vi "Segway - Segue linha suave.vi"() -> ()   [LabVIEW 2016]
uses:
  <vilib>/NXT/Block Support/NXT_InputPort.ctl
  <vilib>/NXT/Subs/MotorOutput.ctl
  <vilib>/NXT/Block Support/NXT_TimerIndex.ctl
  <vilib>/NXT/Block Support/NXT_OutputPort.ctl
  <vilib>/NXT/Dual Mode Library/Waits/Wait_Num.vi
  <vilib>/NXT/Dual Mode Library/Sensors/EV3_Gyro_Reset.vi
  <vilib>/NXT/Dual Mode Library/Motors/ResetMotor.vi
  <vilib>/NXT/Dual Mode Library/Display/drawNumber.vi
  <vilib>/NXT/Dual Mode Library/Sensors/EV3_Color_Reflect.vi
  <vilib>/NXT/Dual Mode Library/Sensors/EV3_Gyro_Rate.vi
  <vilib>/NXT/Dual Mode Library/Motors/Rotation.vi
  <vilib>/NXT/NXTIO Xnodes/NXTIONodeSubVIs/NXTMoveMotors.vi
  <vilib>/NXT/NXTIO Xnodes/AddressXNode/NXTIOAddress.xnode
  <vilib>/NXT/NXTIO Xnodes/NXTIOXNode/NXTIO.xnode
  <vilib>/NXT/Subs/LVHSConnector.ctl
  <vilib>/NXT/LegoClasses/BrickReference/BrickReference.lvclass
panel:
  out "Seguidor E":dbl
  out "Seguidor D":dbl
  in  "stop":bool
  out "e":dbl
  out "Waveform Chart 2":dbl(graph)
  out "b":dbl
  out "a":dbl
  in  "dt_program_flow":dbl
  out "dt":dbl
  out "timer_time":dbl
  out "EncSum":dbl
  out "VelAngRoda2":dbl(graph)
  out "PosAngRoda2":dbl(graph)
  out "PosAngCorpo2":dbl(graph)
  out "VelAngCorpo2":dbl(graph)
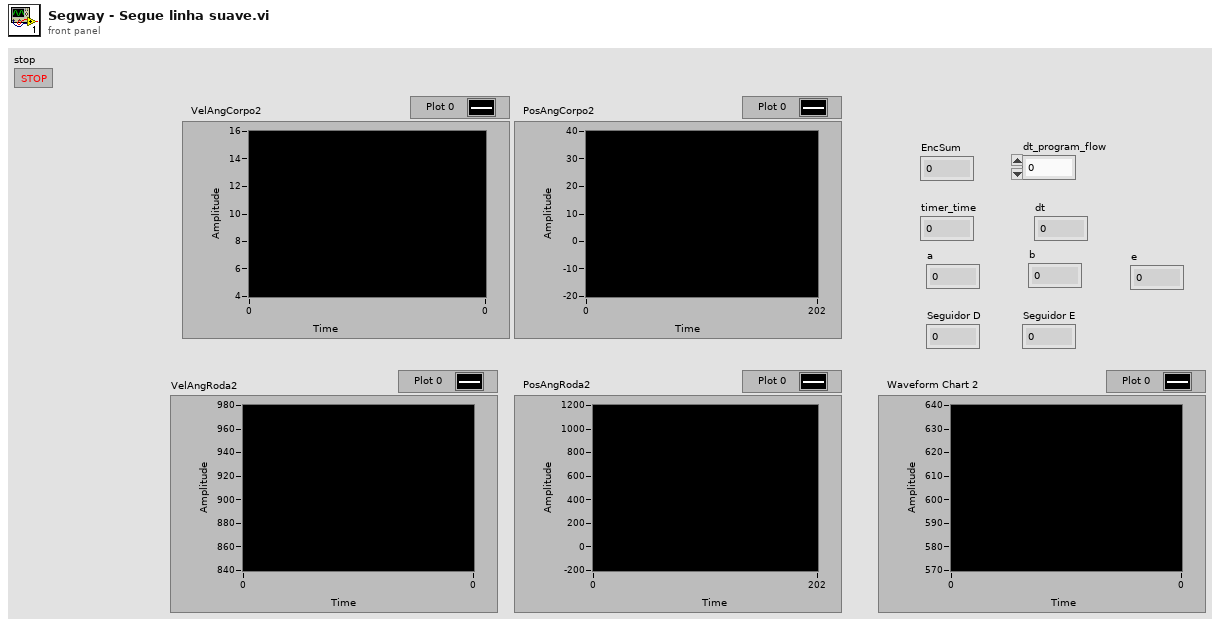
[diagram p1: front panel]
types:
  T1 = typedef "NXT_TimerIndex.ctl" = u8
  T2 = typedef "MotorOutput.ctl" = u8
  T3 = typedef "NXT_InputPort.ctl" = u32
  T4 = typedef "LVHSConnector.ctl" = refnum<class "BrickReference.lvclass">
  T5 = typedef "NXT_OutputPort.ctl" = u8
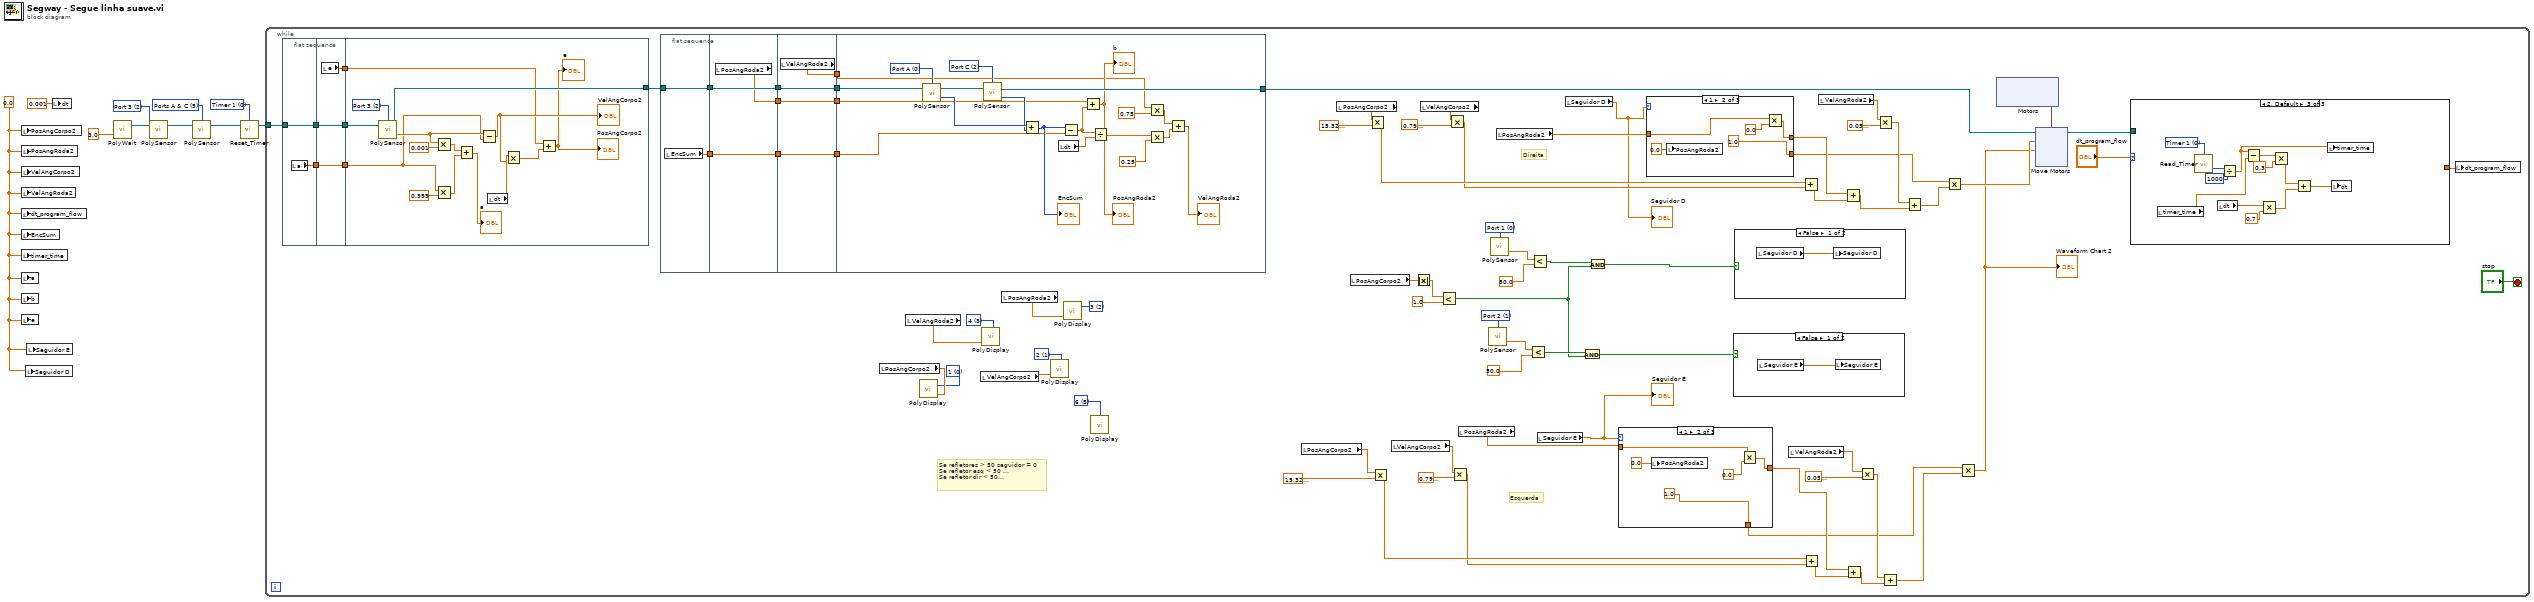
[diagram p0: block diagram]
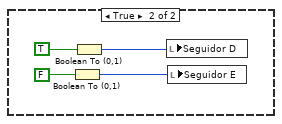
[diagram p2: hidden frame]
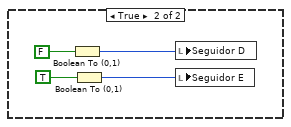
[diagram p3: hidden frame]
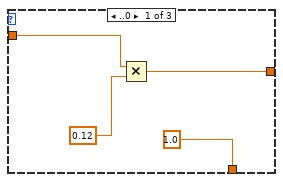
[diagram p4: hidden frame]
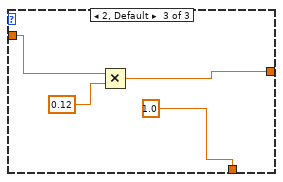
[diagram p5: hidden frame]
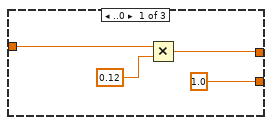
[diagram p6: hidden frame]
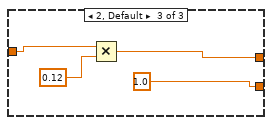
[diagram p7: hidden frame]
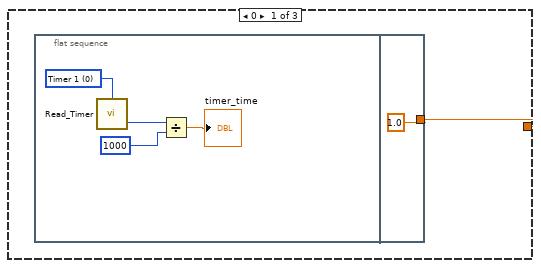
[diagram p8: hidden frame]
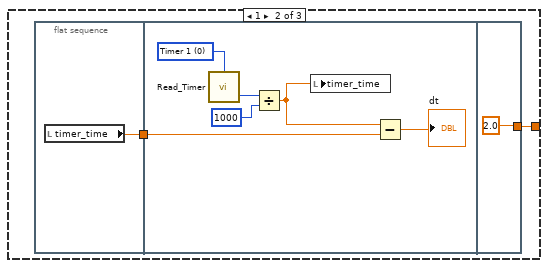
[diagram p9: hidden frame]
diagram:
  w4 = T1 0 items=["Timer 1", "Timer 2", "Timer 3"] ("Timer (Timer 1)")
  w8 = T2 5 items=["Port A"=0, "Port B"=1, "Port C"=2, "Ports A & B"=4, "Ports A & C"=5, "Ports B & C"=6, "All Ports"=3] ("Port (All Ports)")
  w9 = T3 2 items=["Port 1", "Port 2", "Port 3", "Port 4"] ("Port (Port 1)")
  w1 = 0.0 ("PosAngCorpo2")
  n1 = local write "PosAngCorpo2"(w1) -> ()
  n2 = local write "PosAngRoda2"(w1) -> ()
  n3 = local write "VelAngCorpo2"(w1) -> ()
  n4 = local write "VelAngRoda2"(w1) -> ()
  n5 = local write "dt_program_flow"(w1) -> ()
  n6 = local write "EncSum"(w1) -> ()
  n7 = local write "timer_time"(w1) -> ()
  n8 = local write "a"(w1) -> ()
  n9 = local write "b"(w1) -> ()
  n10 = local write "e"(w1) -> ()
  n11 = local write "Seguidor D"(w1) -> ()
  n12 = local write "Seguidor E"(w1) -> ()
  n13 = local write "dt"(0.001 ("dt")) -> ()
  n14 = call-poly <vilib>:"PolyWait.vi"("Time (1 sec)"=sgl 3.0) -> ("NXT/EV3"=w5:T4)  [unwired: 3 in]
  n15 = call-poly <vilib>:"PolySensor.vi"("NXT/EV3"=w5, "Port (Port 1)"=w9) -> ("NXT/EV3"=w7:T4)  [unwired: 2 in]
  n16 = call-poly <vilib>:"PolySensor.vi"("NXT/EV3"=w7, "Port (All Ports)"=w8) -> ("NXT/EV3"=w2:T4)  [unwired: 2 in]
  n17 = call <vilib>:"Reset_Timer.vi"("NXT/EV3"=w2, "Timer (Timer 1)"=w4) -> ("NXT/EV3"=w3:T4)  [unwired: 2 in]
  n18 = while {
    tunnel: w3 -> [w77]
    stop <- "stop" stop-if-true
    w22 = T3 1 items=["Port 1", "Port 2", "Port 3", "Port 4"] ("Port (Port 1)")
    w25 = T3 0 items=["Port 1", "Port 2", "Port 3", "Port 4"] ("Port (Port 1)")
    w26 = i16 5 items=["1", "2", "3", "4", "5", "6", "7", "8", "9", "10", "11", "12"] ("Line")
    w52 = i16 2 items=["1", "2", "3", "4", "5", "6", "7", "8", "9", "10", "11", "12"] ("Line")
    w53 = i16 3 items=["1", "2", "3", "4", "5", "6", "7", "8", "9", "10", "11", "12"] ("Line")
    w54 = i16 1 items=["1", "2", "3", "4", "5", "6", "7", "8", "9", "10", "11", "12"] ("Line")
    w56 = i16 0 items=["1", "2", "3", "4", "5", "6", "7", "8", "9", "10", "11", "12"] ("Line")
    # "Se refletores > 50 seguidor = 0\nSe refletor esq < 50 ...\nSe refletor dir < 50..."
    # "Esquerda"
    # "Direita"
    n19 = flat-sequence {
      tunnel: w77 -> [w156]
      tunnel: [w156] -> w71
      tunnel: [w155] -> w69
      tunnel: w71 -> [w159]
      tunnel: [w159] -> w70
      tunnel: w69 -> [w158]
      tunnel: [w158] -> w68
      tunnel: [w157] -> w67
      tunnel: [w166] -> w80
      tunnel: w70 -> [w162]
      tunnel: w68 -> [w161]
      tunnel: w67 -> [w160]
      frame #0 {
        n20 = local read "a"() -> (w155:dbl)
      }
      frame #1 {
        n21 = local read "e"() -> (w157:dbl)
      }
      frame #2 {
        w170 = T3 2 items=["Port 1", "Port 2", "Port 3", "Port 4"] ("Port (Port 1)")
        n22 = call-poly <vilib>:"PolySensor.vi"("NXT/EV3"=w162, "Port (Port 1)"=w170) -> ("Degrees/Second"=w169:sgl, "NXT/EV3"=w166:T4)  [unwired: 1 in]
        n23 = Multiply(x=w169, y=0.001) -> (x*y=w172:dbl)
        n24 = Multiply(x=w161, y=0.999) -> (x*y=w165:dbl)
        n25 = Add(x=w172, y=w165) -> (x+y=→"a":dbl)
        n26 = Subtract(x=w169, y=w161) -> (x-y=w167:dbl)
        "VelAngCorpo2" <- w167
        n27 = local read "dt"() -> (w168:dbl)
        n28 = Multiply(x=w168, y=w167) -> (x*y=w171:dbl)
        n29 = Add(x=w160, y=w171) -> (x+y=→"PosAngCorpo2" →"e":dbl)
      }
    }
    n30 = flat-sequence {
      tunnel: w80 -> [w127]
      tunnel: [w127] -> w66
      tunnel: [w126] -> w65
      tunnel: w66 -> [w130]
      tunnel: [w130] -> w64
      tunnel: w65 -> [w129]
      tunnel: [w129] -> w62
      tunnel: [w128] -> w59
      tunnel: w64 -> [w134]
      tunnel: [w134] -> w63
      tunnel: w62 -> [w133]
      tunnel: [w133] -> w61
      tunnel: [w132] -> w60
      tunnel: w59 -> [w131]
      tunnel: [w131] -> w58
      tunnel: w63 -> [w143]
      tunnel: [w141] -> w79
      tunnel: w61 -> [w137]
      tunnel: w60 -> [w136]
      tunnel: w58 -> [w135]
      frame #0 {
        n31 = local read "EncSum"() -> (w126:dbl)
      }
      frame #1 {
        n32 = local read "PosAngRoda2"() -> (w128:dbl)
      }
      frame #2 {
        n33 = local read "VelAngRoda2"() -> (w132:dbl)
      }
      frame #3 {
        w145 = T5 2 items=["Port A", "Port B", "Port C", "Port D"] ("Port (Port A)")
        w148 = T5 0 items=["Port A", "Port B", "Port C", "Port D"] ("Port (Port A)")
        n34 = call-poly <vilib>:"PolySensor.vi"("NXT/EV3"=w143, "Port (Port A)"=w148) -> ("Angle of Rotation"=w147:i32, "NXT/EV3"=w142:T4)  [unwired: 1 in]
        n35 = call-poly <vilib>:"PolySensor.vi"("NXT/EV3"=w142, "Port (Port A)"=w145) -> ("Angle of Rotation"=w144:i32, "NXT/EV3"=w141:T4)  [unwired: 1 in]
        n36 = Add(x=w147, y=w144) -> (x+y=w154:i32)
        "EncSum" <- w154
        n37 = local read "dt"() -> (w146:dbl)
        n38 = Subtract(x=w154, y=w137) -> (x-y=w153:dbl)
        n39 = Add(x=w135, y=w153) -> (x+y=→"PosAngRoda2" →"b":dbl)
        n40 = Divide(x=w153, y=w146) -> (x/y=w149:dbl)
        n41 = Multiply(x=w136, y=0.75) -> (x*y=w139:dbl)
        n42 = Multiply(x=w149, y=sgl 0.25) -> (x*y=w151:dbl)
        n43 = Add(x=w139, y=w151) -> (x+y=→"VelAngRoda2":dbl)
      }
    }
    n44 = local read "PosAngCorpo2"() -> (w57:dbl)
    n45 = local read "VelAngRoda2"() -> (w50:dbl)
    n46 = call-poly <vilib>:"PolyDisplay.vi"("number"=w57, "Line"=w56) -> ()  [unwired: 2 in, 1 out]
    n47 = local read "VelAngCorpo2"() -> (w55:dbl)
    n48 = call-poly <vilib>:"PolyDisplay.vi"("number"=w50, "Line"=w53) -> ()  [unwired: 2 in, 1 out]
    n49 = local read "PosAngRoda2"() -> (w51:dbl)
    n50 = call-poly <vilib>:"PolyDisplay.vi"("number"=w55, "Line"=w54) -> ()  [unwired: 2 in, 1 out]
    n51 = call-poly <vilib>:"PolyDisplay.vi"("number"=w51, "Line"=w52) -> ()  [unwired: 2 in, 1 out]
    n52 = call-poly <vilib>:"PolyDisplay.vi"("Line"=w26) -> ()  [unwired: 3 in, 1 out]
    n53 = local read "PosAngCorpo2"() -> (w34:dbl)
    n54 = local read "PosAngCorpo2"() -> (w83:dbl)
    n55 = local read "PosAngCorpo2"() -> (w29:dbl)
    n56 = Multiply(x=w83, y=sgl 15.33) -> (x*y=w76:dbl)
    n57 = Multiply(x=w34, y=sgl 15.33) -> (x*y=w41:dbl)
    n58 = local read "VelAngCorpo2"() -> (w35:dbl)
    n59 = Absolute Value(x=w29) -> (abs(x)=w28:dbl)
    n60 = local read "VelAngCorpo2"() -> (w82:dbl)
    n61 = Less?(x=w28, y=1.0) -> (x < y?=w15:bool)
    n62 = Multiply(x=w82, y=sgl 0.79) -> (x*y=w75:dbl)
    n63 = Multiply(x=w35, y=sgl 0.79) -> (x*y=w40:dbl)
    n64 = local read "PosAngRoda2"() -> (w32:dbl)
    n65 = call-poly <vilib>:"PolySensor.vi"("Port (Port 1)"=w22) -> ("Scaled Value"=w21:sgl)  [unwired: 2 in, 1 out]
    n66 = call-poly <vilib>:"PolySensor.vi"("Port (Port 1)"=w25) -> ("Scaled Value"=w24:sgl)  [unwired: 2 in, 1 out]
    n67 = local read "PosAngRoda2"() -> (w48:dbl)
    n68 = Less?(x=w21, y=50.0) -> (x < y?=w17:bool)
    n69 = Less?(x=w24, y=50.0) -> (x < y?=w19:bool)
    n70 = local read "Seguidor E"() -> (w11:dbl)
    "Seguidor E" <- w11
    n71 = local read "Seguidor D"() -> (w12:dbl)
    "Seguidor D" <- w12
    n72 = And(x=w17, y=w15) -> (x .and. y?=w16:bool)
    n73 = And(x=w19, y=w15) -> (x .and. y?=w18:bool)
    n74 = case shown="1" w11 {
      tunnel: w32 -> [w102 w106 w111]
      tunnel: [w101 w105 w110] -> w31
      tunnel: [1.0 ("y") 1.0 ("y") 1.0 ("y")] -> w30
      frame ..0 {
        n75 = Multiply(x=w102, y=0.12) -> (x*y=w101:dbl)
      }
      frame 1 {
        n76 = local write "PosAngRoda2"(0.0) -> ()
        n77 = Multiply(x=w106, y=0.0) -> (x*y=w105:dbl)
      }
      frame 2, Default {
        n78 = Multiply(x=w111, y=0.12) -> (x*y=w110:dbl)
      }
    }
    n79 = case shown="1" w12 {
      tunnel: w48 -> [w116 w120 w124]
      tunnel: [w114 w119 w123] -> w47
      tunnel: [1.0 ("y") 1.0 ("y") 1.0 ("y")] -> w46
      frame ..0 {
        n80 = Multiply(x=w116, y=0.12) -> (x*y=w114:dbl)
      }
      frame 1 {
        n81 = local write "PosAngRoda2"(0.0 ("PosAngRoda2")) -> ()
        n82 = Multiply(x=w120, y=0.0) -> (x*y=w119:dbl)
      }
      frame 2, Default {
        n83 = Multiply(x=w124, y=0.12) -> (x*y=w123:dbl)
      }
    }
    n84 = case shown="False" w16 {
      frame False {
        n85 = local read "Seguidor E"() -> (w90:dbl)
        n86 = local write "Seguidor E"(w90) -> ()
      }
      frame True {
        n87 = Boolean To (0,1)(Boolean=FALSE) -> (0, 1=w93:i16)
        n88 = Boolean To (0,1)(Boolean=TRUE) -> (0, 1=w91:i16)
        n89 = local write "Seguidor D"(w91) -> ()
        n90 = local write "Seguidor E"(w93) -> ()
      }
    }
    n91 = case shown="False" w18 {
      frame False {
        n92 = local read "Seguidor D"() -> (w95:dbl)
        n93 = local write "Seguidor D"(w95) -> ()
      }
      frame True {
        n94 = Boolean To (0,1)(Boolean=FALSE) -> (0, 1=w98:i16)
        n95 = Boolean To (0,1)(Boolean=TRUE) -> (0, 1=w96:i16)
        n96 = local write "Seguidor D"(w98) -> ()
        n97 = local write "Seguidor E"(w96) -> ()
      }
    }
    n98 = local read "VelAngRoda2"() -> (w33:dbl)
    n99 = Add(x=w76, y=w75) -> (x+y=w74:dbl)
    n100 = Add(x=w41, y=w40) -> (x+y=w39:dbl)
    n101 = local read "VelAngRoda2"() -> (w81:dbl)
    n102 = Add(x=w47, y=w74) -> (x+y=w73:dbl)
    n103 = Add(x=w31, y=w39) -> (x+y=w38:dbl)
    n104 = Multiply(x=w33, y=sgl 0.06) -> (x*y=w37:dbl)
    n105 = Multiply(x=w81, y=sgl 0.06) -> (x*y=w72:dbl)
    n106 = Add(x=w37, y=w38) -> (x+y=w36:dbl)
    n107 = Add(x=w72, y=w73) -> (x+y=w45:dbl)
    n108 = Multiply(x=w46, y=w45) -> (x*y=w14:dbl)
    n109 = Multiply(x=w30, y=w36) -> (x*y=w13:dbl)
    "Waveform Chart 2" <- w13
    n110 = xnode "Motors"() -> ("Motor"=w87:cluster{"Port":T5, "Port":T5})
    n111 = xnode "Move Motors"("Power/Speed 2"=w13, "Power/Speed 1"=w14, "Motors"=w87, "NXT/EV3"=w79) -> ("NXT/EV3"=w78:T4)
    n112 = case shown="2, Default" "dt_program_flow" {
      tunnel: [w184 w190 _] -> w89
      tunnel: w78 -> [_ _ _]
      frame 0 {
        n113 = flat-sequence {
          tunnel: [1.0 ("dt_program_flow")] -> w184
          frame #0 {
            w188 = T1 0 items=["Timer 1", "Timer 2", "Timer 3"] ("Timer (Timer 1)")
            n114 = call <vilib>:"Read_Timer.vi"("Timer (Timer 1)"=w188) -> ("Value (msec)"=w185:u32)  [unwired: 2 in, 1 out]
            n115 = Divide(x=w185, y=u32 1000) -> (x/y=→"timer_time":dbl)
          }
          frame #1 {
          }
        }
      }
      frame 1 {
        n116 = flat-sequence {
          tunnel: [w192] -> w191
          tunnel: w191 -> [w198]
          tunnel: [2.0 ("dt_program_flow")] -> w190
          frame #0 {
            n117 = local read "timer_time"() -> (w192:dbl)
          }
          frame #1 {
            w196 = T1 0 items=["Timer 1", "Timer 2", "Timer 3"] ("Timer (Timer 1)")
            n118 = call <vilib>:"Read_Timer.vi"("Timer (Timer 1)"=w196) -> ("Value (msec)"=w195:u32)  [unwired: 2 in, 1 out]
            n119 = Divide(x=w195, y=u32 1000) -> (x/y=w193:dbl)
            n120 = local write "timer_time"(w193) -> ()
            n121 = Subtract(x=w193, y=w198) -> (x-y=→"dt":dbl)
          }
          frame #2 {
          }
        }
      }
      frame 2, Default {
        w203 = T1 0 items=["Timer 1", "Timer 2", "Timer 3"] ("Timer (Timer 1)")
        n122 = local read "timer_time"() -> (w200:dbl)
        n123 = call <vilib>:"Read_Timer.vi"("Timer (Timer 1)"=w203) -> ("Value (msec)"=w202:u32)  [unwired: 2 in, 1 out]
        n124 = local read "dt"() -> (w205:dbl)
        n125 = Divide(x=w202, y=u32 1000) -> (x/y=w210:dbl)
        n126 = Subtract(x=w210, y=w200) -> (x-y=w209:dbl)
        n127 = Multiply(x=w205, y=0.7) -> (x*y=w204:dbl)
        n128 = Multiply(x=w209, y=0.3) -> (x*y=w207:dbl)
        n129 = Add(x=w207, y=w204) -> (x+y=w211:dbl)
        n130 = local write "timer_time"(w210) -> ()
        n131 = local write "dt"(w211) -> ()
      }
    }
    n132 = local write "dt_program_flow"(w89) -> ()
  }
